vi "Add channel1553.vi"(6 "channel1553 configuration":T1={"channelBufferMaxSizeKB"=1024, "amplitudeAdjustEnable"=FALSE, "amplitudePercent"=50.0, "termination"=0, "modeCodes"=0, "broadcast"=FALSE} {"termination" items=["Off", "OnA", "OnB", "On"]; "modeCodes" items=["MC01", "MC1", "MC0", "None"]}, 7 "errorInjection configuration":T2 {"errorMessages" items=["Tagged", "Any"]; "state" items=["Off", "On", "Once", "External"]}, 8 "error in":errorcluster, 9 "hardwareChannel (-1)":i32=-1, 10 "name":string, 11 "xml ref in":refnum<k24>) -> (0 "error out":errorcluster, 2 "new channel1553 out":refnum<k24>, 3 "xml ref out":refnum<k24>)   [LabVIEW 2020, in "Ballard_1553_Hardware_ni.lvlib"]
uses:
  Ballard_1553_Hardware_ni.lvlib
  C:/Users/Administrator/Desktop/GIT/Ballard-MIL-STD-1553-Custom-Device/Source/System Explorer/SubVIs/Parse XML Ballard/1.2/BTIXML_SerDes.dll
  Ballard-MIL-STD-1553-Custom-Device/Source/System Explorer/SubVIs/Parse XML Ballard/1.2/BTIXML_SerDes.dll
  _typedefs/channel1553_errorInjection_type.ctl
  _typedefs/channel1553_type.ctl
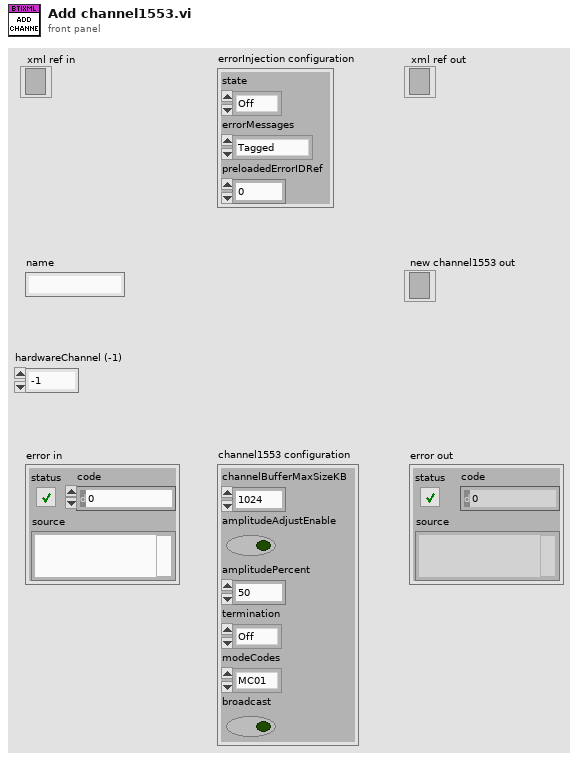
[diagram p1: front panel]
types:
  T1 = typedef "Ballard_1553_Hardware_ni.lvlib/channel1553_type.ctl" = cluster{"channelBufferMaxSizeKB":u32, "amplitudeAdjustEnable":bool, "amplitudePercent":dbl, "termination":i32, "modeCodes":i32, "broadcast":bool}
  T2 = typedef "Ballard_1553_Hardware_ni.lvlib/channel1553_errorInjection_type.ctl" = cluster{"state":i32, "errorMessages":i32, "preloadedErrorIDRef":i32}
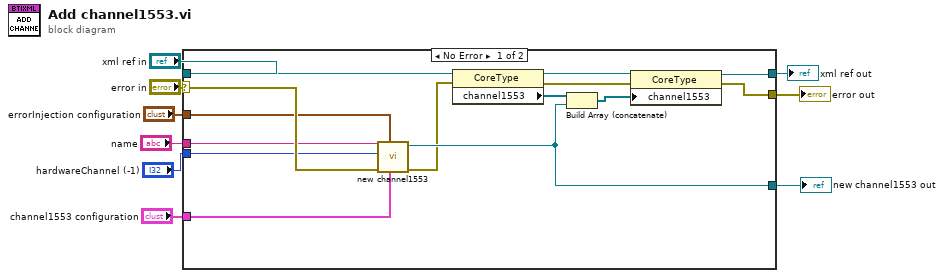
[diagram p0: block diagram]
diagram:
  n1 = case shown="No Error" "error in" {
    selector: "error in" -> [w15 w24]
    tunnel: [w21 w24] -> w9
    tunnel: [w19 w25] -> w8
    tunnel: "xml ref in" -> [w23 w25]
    tunnel: [w16 _] -> w5
    tunnel: "name" -> [w13 _]
    tunnel: "errorInjection configuration" -> [w12 _]
    tunnel: "hardwareChannel (-1)" -> [w11 _]
    tunnel: "channel1553 configuration" -> [w10 _]
    frame No Error {
      n2 = call "new channel1553.vi"("channel1553 configuration"=w10, "errorInjection configuration"=w12, "error in"=w15, "hardwareChannel (-1)"=w11, "name"=w13) -> ("error out"=w14:errorcluster, "new channel1553"=w16:refnum<k24>)  [unwired: 5 in]
      n3 = property class="CoreType"(reference=w23, error in=w14) -> (reference out=w20:refnum<k24>, error out=w18:errorcluster, "channel1553"=w22:refnum<k24>[])
      n4 = Build Array (concatenate)(w22, w16) -> (w17:refnum<k24>[])
      n5 = property class="CoreType"(reference=w20, error in=w18, "channel1553"=w17) -> (reference out=w19:refnum<k24>, error out=w21:errorcluster)
    }
    frame Error {
    }
  }
  "error out" <- w9
  "xml ref out" <- w8
  "new channel1553 out" <- w5
